vi "DrawItemsDynamic.vi"(8 "error in (no error)":errorcluster, 11 "OrderSelection in":refnum<class "OrderSelection.lvclass">) -> (0 "error out":errorcluster, 3 "OrderSelection out":refnum<class "OrderSelection.lvclass">)   [LabVIEW 2020, in "OrderSelection.lvclass"]
uses:
  OrderSelection.lvclass
  OrderSelection.lvclass/OrderSelection.ctl
  Read Items.vi
  Read SelectedItem.vi
  Read ItemGraphic.vi
  Read PositionIndex.vi
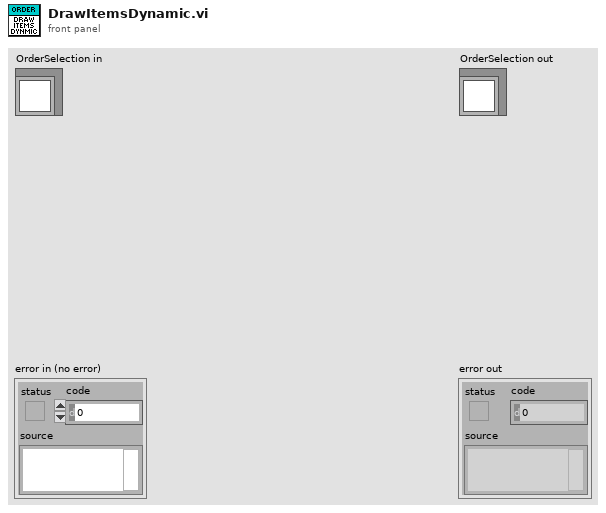
[diagram p1: front panel]
types:
  T1 = cluster{"horizontal":enum16{"left", "center", "right"}, "vertical":enum16{"top", "center", "bottom"}}
  T2 = cluster{"Horizontal Shift":i16, "Vertical Shift":i16}
  T3 = cluster{"Width":i16, "Style":enum32{"Solid", "Dash", "Dot", "DashDot", "DashDotDot"}}
  T4 = cluster{"left":i16, "top":i16, "right":i16, "bottom":i16}
  T5 = typedef "imagedata.ctl" = cluster{"image type":i32, "image depth":i32, "image":u8[], "mask":u8[], "colors":u32[], "Rectangle":cluster{"left":i16, "top":i16, "right":i16, "bottom":i16}}
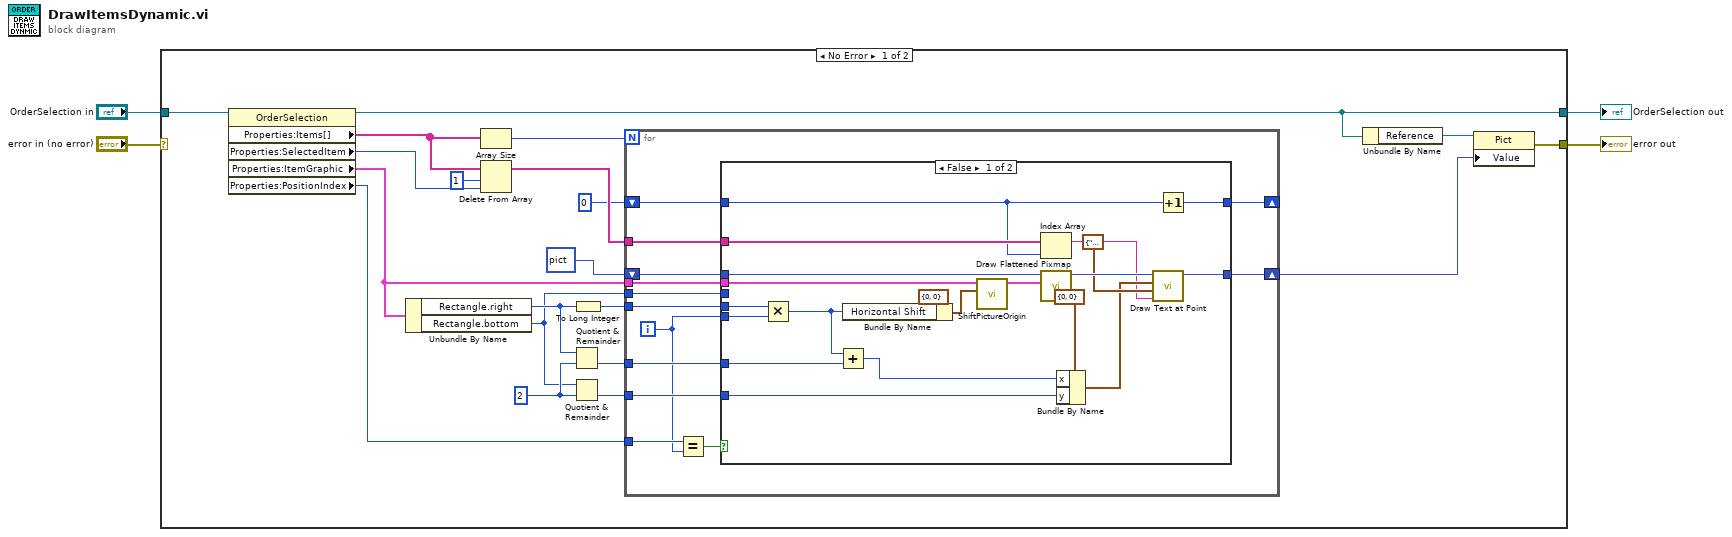
[diagram p0: block diagram]
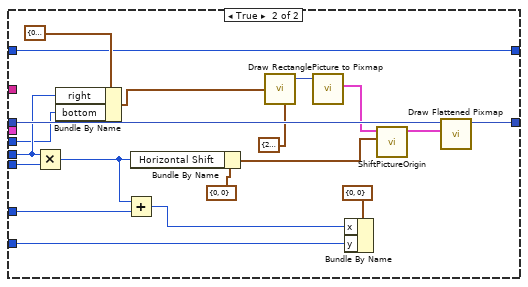
[diagram p2: hidden frame]
diagram:
  n1 = case shown="No Error" "error in (no error)" {
    selector: "error in (no error)" -> [_ w78]
    tunnel: [w15 w78] -> w3
    tunnel: [w14 w77] -> w1
    tunnel: "OrderSelection in" -> [w18 w77]
    frame No Error {
      w21 = i16 2 ("y")
      n2 = property class="OrderSelection"(reference=w18) -> (reference out=w14:refnum<class "OrderSelection.lvclass">, "Properties:Items[]"=w10:string[], "Properties:SelectedItem"=w7:i32, "Properties:ItemGraphic"=w13:T5, "Properties:PositionIndex"=w5:i32)  [unwired: 1 in, 1 out]
      n3 = Unbundle By Name(w13) -> ("Rectangle.right"=w22:i16, "Rectangle.bottom"=w12:i16)
      n4 = Array Size(array=w10) -> (size(s)=w9:i32)
      n5 = Delete From Array(array=w10, length=1, index=w7) -> (array with subset deleted=w11:string[])  [unwired: 1 out]
      n6 = Quotient & Remainder(x=w22, y=w21) -> (floor(x/y)=w20:i16)  [unwired: 1 out]
      n7 = Quotient & Remainder(x=w12, y=w21) -> (floor(x/y)=w19:i16)  [unwired: 1 out]
      n8 = To Long Integer(number=w22) -> (32bit integer=w23:i32)
      n9 = for {
        N: w9 -> [_]
        tunnel: w13 -> [w37]
        shift-right: [w34] -> w16
        shift-left: picture data[5B] ("new picture") -> [w36]
        tunnel: w23 -> [w35]
        tunnel: w20 -> [w32]
        tunnel: w19 -> [w33]
        tunnel: w11 -> [w31]
        tunnel: w5 -> [w30]
        tunnel: w12 -> [w28]
        shift-right: [w26] -> _
        shift-left: 0 -> [w27]
        i -> [w25]
        n10 = Equal?(x=w30, y=w25) -> (x = y?=w29:bool)
        n11 = case shown="False" w29 {
          tunnel: w37 -> [w55 _]
          tunnel: w36 -> [w52 w74]
          tunnel: w35 -> [w51 w65]
          tunnel: [w50 w76] -> w34
          tunnel: w33 -> [w43 w70]
          tunnel: w32 -> [w46 w72]
          tunnel: w31 -> [w44 _]
          tunnel: w28 -> [_ w64]
          tunnel: w27 -> [w41 w60]
          tunnel: [w40 w60] -> w26
          tunnel: w25 -> [w38 w58]
          frame False {
            n12 = Multiply(x=w51, y=w38) -> (x*y=w39:i32)
            n13 = Add(x=w39, y=w46) -> (x+y=w45:i32)
            n14 = Bundle By Name(cluster=T2 {"Horizontal Shift"=0, "Vertical Shift"=0} ("Shift(0, 0)"), "Horizontal Shift"=w39) -> (w53:T2)
            n15 = call "ShiftPictureOrigin.vi"("Shift(0, 0)"=w53, "image data IN"=w55) -> ("image data OUT"=w57:T5)  [unwired: 8 in, 1 out]
            n16 = Index Array(array=w44, index=w41) -> (element=w42:string)
            n17 = call <vilib>:"Draw Flattened Pixmap.vi"("image data"=w57, "picture"=w52) -> ("new picture"=w56:picture)  [unwired: 7 in]
            n18 = Bundle By Name(cluster=cluster{"x":i16, "y":i16} {"x"=0, "y"=0} ("origin"), "x"=w45, "y"=w43) -> (w47:cluster{"x":i16, "y":i16})
            n19 = call <vilib>:"Draw Text at Point.vi"("text"=w42, "alignment(left, top)"=T1 {"horizontal"=enum."center", "vertical"=enum."center"}, "origin"=w47, "picture"=w56) -> ("new picture"=w50:picture)  [unwired: 6 in, 1 out]
            n20 = Increment(x=w41) -> (x+1=w40:i32)
          }
          frame True {
            n21 = Multiply(x=w65, y=w58) -> (x*y=w59:i32)
            n22 = Bundle By Name(cluster=T4 {"left"=0, "top"=0, "right"=0, "bottom"=0} ("rect"), "right"=w65, "bottom"=w64) -> (w62:T4)
            n23 = Add(x=w59, y=w72) -> (x+y=w71:i32)
            n24 = Bundle By Name(cluster=T2 {"Horizontal Shift"=0, "Vertical Shift"=0} ("Shift(0, 0)"), "Horizontal Shift"=w59) -> (w68:T2)
            n25 = call <vilib>:"Draw Rectangle.vi"("rect"=w62, "pen"=T3 {"Width"=2, "Style"=enum."Dot"}) -> ("new picture"=w61:picture)  [unwired: 7 in]
            n26 = call <vilib>:"Picture to Pixmap.vi"("picture"=w61) -> ("image data"=w67:T5)  [unwired: 9 in, 1 out]
            n27 = Bundle By Name(cluster=cluster{"x":i16, "y":i16} {"x"=0, "y"=0} ("origin"), "x"=w71, "y"=w70) -> ()  [unwired: 1 out]
            n28 = call "ShiftPictureOrigin.vi"("Shift(0, 0)"=w68, "image data IN"=w67) -> ("image data OUT"=w69:T5)  [unwired: 8 in, 1 out]
            n29 = call <vilib>:"Draw Flattened Pixmap.vi"("image data"=w69, "picture"=w74) -> ("new picture"=w76:picture)  [unwired: 7 in]
          }
        }
      }
      n30 = Unbundle By Name(w14) -> ("Reference"=w17:refnum<vi>)
      n31 = property class="Pict"(reference=w17, "Value"=w16) -> (error out=w15:errorcluster)  [unwired: 1 in, 1 out]
    }
    frame Error {
    }
  }
  "error out" <- w3
  "OrderSelection out" <- w1
